vi "output.vi"(1 "C":bool, 2 "OVERFLOW":bool, 3 "INPUT":T2, 4 "R":bool) -> (0 "OUTPUT":T1)   [LabVIEW 2013]
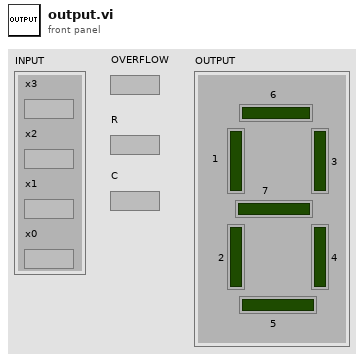
[diagram p1: front panel]
types:
  T1 = cluster{"6":bool, "3":bool, "1":bool, "7":bool, "2":bool, "4":bool, "5":bool}
  T2 = cluster{"x3":bool, "x2":bool, "x1":bool, "x0":bool}
  T3 = cluster{"y3":bool, "y2":bool, "y1":bool, "y0":bool}
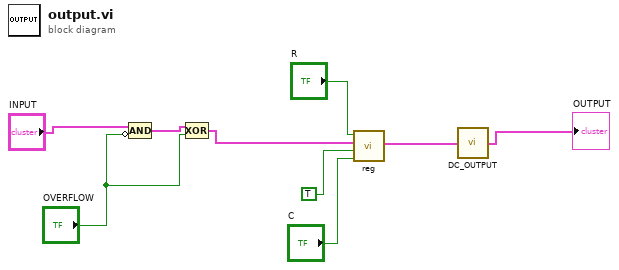
[diagram p0: block diagram]
diagram:
  n1 = Compound Arithmetic op=AND("INPUT", invert "OVERFLOW") -> (w3:T2)
  n2 = Compound Arithmetic op=XOR(w3, "OVERFLOW") -> (w2:T2)
  n3 = call "reg.vi"("C"="C", "WRITE"=TRUE, "INPUT"=w2, "R"="R") -> ("OUTPUT"=w9:T3)
  n4 = call "DC_OUTPUT.vi"("INPUT"=w9) -> ("OUTPUT"=→"OUTPUT":T1)
